vi "RTS Read Data File.vi"(8 "Error In":errorcluster, 9 "Full Item Names":string[](array[string]), 10 "Index Locations":i32[](array[numeric]), 11 "File Location":path) -> (0 "Error Out":errorcluster, 3 "Correctly Indexed Array":dbl[][](array[numeric]))   [LabVIEW 2016]
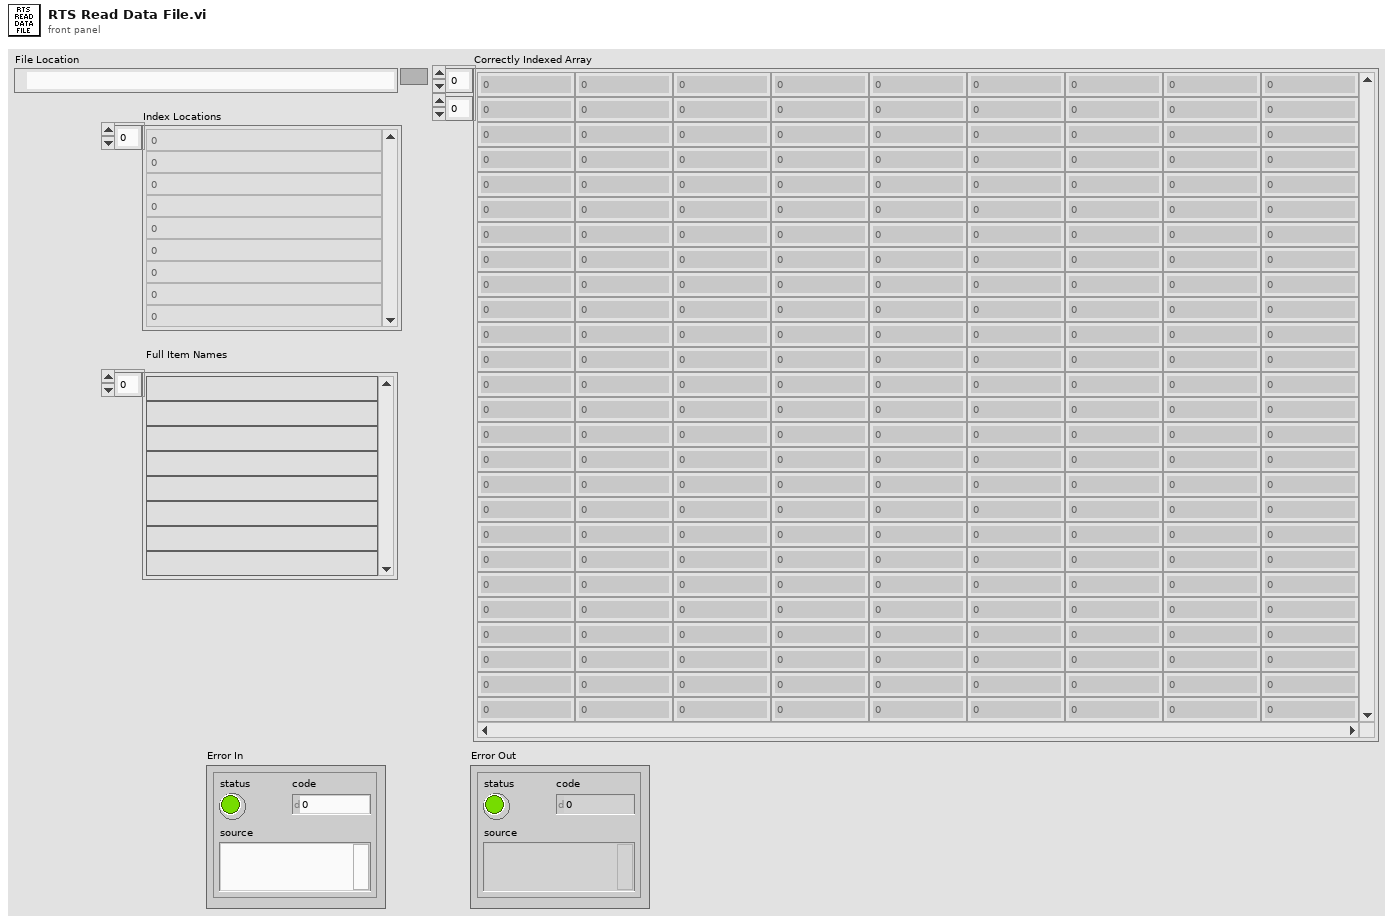
[diagram p1: front panel]
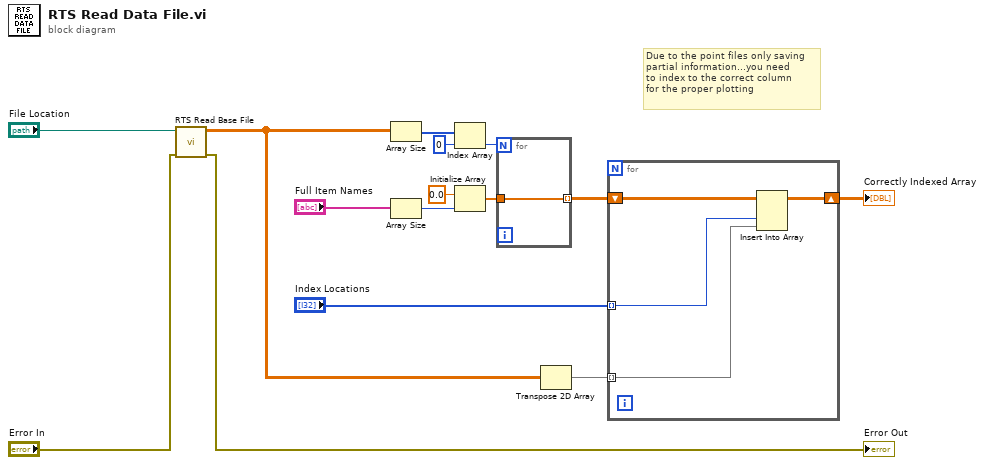
[diagram p0: block diagram]
diagram:
  # "Due to the point files only saving\npartial information...you need\nto index to the correct column \nfor the proper plotting"
  n1 = call "RTS Read Base File.vi"("Error In"="Error In", "File Location"="File Location") -> ("Error Out"=→"Error Out":errorcluster, "all rows"=w3:dbl[][])  [unwired: 8 in]
  n2 = Array Size(array=w3) -> (size(s)=w8:i32[])
  n3 = Array Size(array="Full Item Names") -> (size(s)=w9:i32)
  n4 = Index Array(array=w8, index=0) -> (element=w5:i32)
  n5 = Initialize Array(0.0 ("element"), w9) -> (w6:dbl[])
  n6 = for {
    N: w5 -> [_]
    tunnel: w6 -> [w16]
    tunnel: [w16] -> w12 mode=indexing
  }
  n7 = Transpose 2D Array(2D array=w3) -> (transposed array=w4:dbl[][])
  n8 = for {
    tunnel: w4 -> [w18] mode=indexing
    tunnel: "Index Locations" -> [w19] mode=indexing
    shift-right: [w17] -> w14
    shift-left: w12 -> [w20]
    n9 = Insert Into Array(array=w20, index (col)=w19, new element=w18) -> (w17:dbl[][])  [unwired: 1 in]
  }
  "Correctly Indexed Array" <- w14
